vi "To string.vi"(8 "error in (no error)":errorcluster, 11 "Power control in":refnum<class "Power control.lvclass">) -> (0 "error out":errorcluster, 2 "String":string, 3 "Power control out":refnum<class "Power control.lvclass">)   [LabVIEW 2018, in "Power control.lvclass"]
uses:
  Power control.lvclass
  Power control.lvclass/Power control.ctl
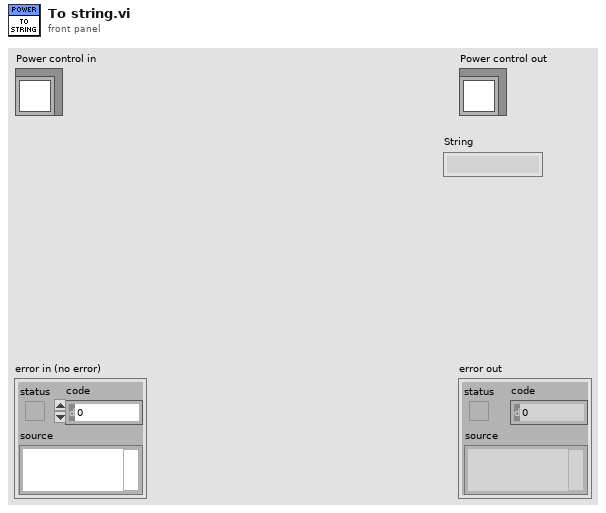
[diagram p1: front panel]
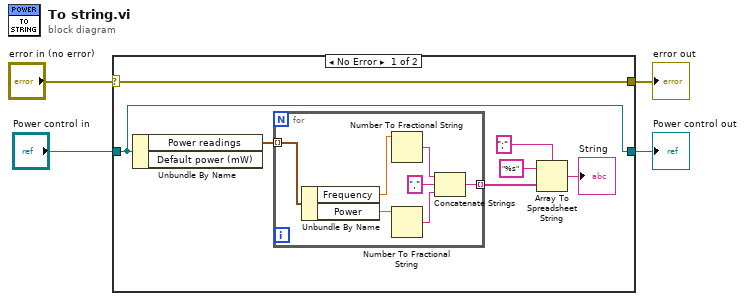
[diagram p0: block diagram]
diagram:
  n1 = case shown="No Error" "error in (no error)" {
    selector: "error in (no error)" -> [w11 w20]
    tunnel: [w11 w20] -> w3
    tunnel: [w10 w19] -> w1
    tunnel: "Power control in" -> [w10 w19]
    frame No Error {
      n2 = Unbundle By Name(w10) -> ("Power readings"=w9:cluster{"Frequency":dbl, "Power":dbl}[])  [unwired: 1 out]
      n3 = for {
        tunnel: w9 -> [w18] mode=indexing
        tunnel: [w12] -> w8 mode=indexing
        n4 = Unbundle By Name(w18) -> ("Frequency"=w17:dbl, "Power"=w16:dbl)
        n5 = Number To Fractional String(number=w17) -> (F-format string=w15:string)  [unwired: 3 in]
        n6 = Number To Fractional String(number=w16) -> (F-format string=w14:string)  [unwired: 3 in]
        n7 = Concatenate Strings(w15, ",", w14) -> (w12:string)
      }
      n8 = Array To Spreadsheet String(delimiter (Tab)=";", array=w8, 3:"%s" ("format string")) -> (spreadsheet string=→"String":string)
    }
    frame Error {
    }
  }
  "error out" <- w3
  "Power control out" <- w1
